vi "Attach Observer (polymorphic).vi"   [LabVIEW 2011, in "Messenging.lvlib"]
uses:
  Messenging.lvlib
  Parallel Process/Parallel Process.lvclass
  Messenger (Parent)/MGR.lvclass
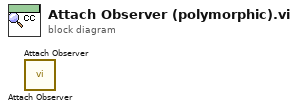
[diagram p0: block diagram]
diagram:
  n1 = call "Attach Observer.vi"() -> ()  [unwired: 11 in, 1 out]
  n2 = call "Attach Observer.vi"() -> ()  [unwired: 11 in, 1 out]
